vi "execute.vi"(8 "error in (no error)":errorcluster, 9 "data collection in":refnum<class "GenericComponent.lvclass">, 10 "imaging mode in":refnum<class "GenericComponent.lvclass">, 11 "adapter in":refnum<class "AdapterMG090709ImagingModeToDataCollection.lvclass">) -> (0 "error out":errorcluster, 1 "data collection out":refnum<class "GenericComponent.lvclass">, 2 "imaging mode out":refnum<class "GenericComponent.lvclass">, 3 "adapter out":refnum<class "AdapterMG090709ImagingModeToDataCollection.lvclass">)   [LabVIEW 2010, in "AdapterMG090709ImagingModeToDataCollection.lvclass"]
uses:
  AdapterMG090709ImagingModeToDataCollection.lvclass
  common/classes/GenericComponent/GenericComponent/GenericComponent.lvclass
  ImagingMode/ImagingModeMG090624Camera/ImagingModeMG090624Camera/ImagingModeMG090624Camera.lvclass
  DataCollection/DataCollectionDL090215/DataCollectionDL090215/DataCollectionDL090215.lvclass
panel:
  # "imaging mode: ImagingModeMG090624Camera\ndata collection: DataCollectionDL090215"
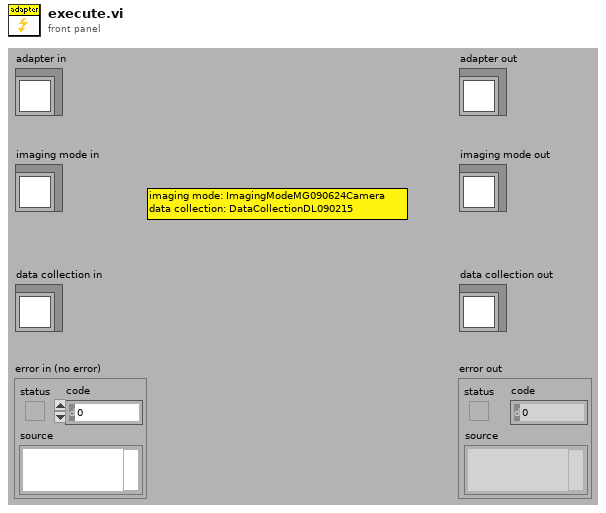
[diagram p1: front panel]
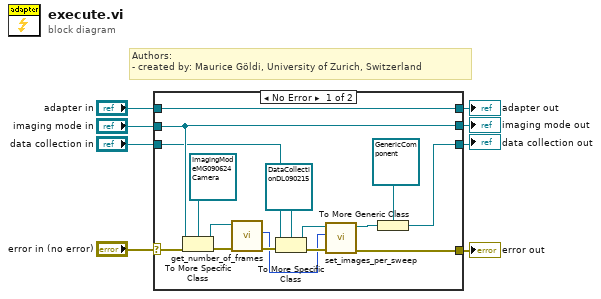
[diagram p0: block diagram]
diagram:
  # "Authors: \n- created by: Maurice Göldi, University of Zurich, Switzerland"
  n1 = case shown="No Error" "error in (no error)" {
    selector: "error in (no error)" -> [w24 w25]
    tunnel: "imaging mode in" -> [w23 w28]
    tunnel: [w23 w28] -> w6
    tunnel: [w22 w27] -> w5
    tunnel: "adapter in" -> [w22 w27]
    tunnel: "data collection in" -> [w18 w26]
    tunnel: [w16 w26] -> w2
    tunnel: [w10 w25] -> w1
    frame No Error {
      n2 = To More Specific Class(target class=refnum<class "ImagingModeMG090624Camera.lvclass"> refnum ("ScanModeMG090624Camera.lvclass"), reference=w23, error in=w24) -> (specific class reference=w21:refnum<class "ImagingModeMG090624Camera.lvclass">, error out=w20:errorcluster)
      n3 = call-dynamic "get_number_of_frames.vi"("error in (no error)"=w20, "ScanModeMG090624Camera in"=w21) -> ("error out"=w19:errorcluster, "number of frames"=w13:i32)  [unwired: 7 in, 1 out]
      n4 = To More Specific Class(target class=refnum<class "DataCollectionDL090215.lvclass"> refnum ("DataCollectionDL090215.lvclass"), reference=w18, error in=w19) -> (specific class reference=w12:refnum<class "DataCollectionDL090215.lvclass">, error out=w14:errorcluster)
      n5 = call "set_images_per_sweep.vi"("error in (no error)"=w14, "images per sweep"=w13, "DataCollectionDL090215 in"=w12) -> ("error out"=w10:errorcluster, "DataCollectionDL090215 out"=w11:refnum<class "DataCollectionDL090215.lvclass">)  [unwired: 7 in]
      n6 = To More Generic Class(target class=refnum<class "GenericComponent.lvclass"> refnum ("GenericComponent.lvclass"), reference=w11) -> (generic class reference=w16:refnum<class "GenericComponent.lvclass">)
    }
    frame Error {
    }
  }
  "error out" <- w1
  "adapter out" <- w5
  "imaging mode out" <- w6
  "data collection out" <- w2
